vi "Day 8 Task 1.vi"() -> ()   [LabVIEW 2018]
uses:
  <userlib>/_OpenG.lib/array/array.llb/Search 1D Array (I32)__ogtk.vi
  <userlib>/_OpenG.lib/array/array.llb/Delete Elements from 1D Array (I32)__ogtk.vi
  <userlib>/_OpenG.lib/array/array.llb/Remove Duplicates from 1D Array (String)__ogtk.vi
panel:
  out "and the other is f":string
  out "the letter it doesn't have is c":string
  out "6":string
  out "representation of cf":string
  out "representation of eg":string
  out "representation of bd":string
  out "representation of a":string
  out "Found? (index is digit)":bool[][](array[boolean])
  out "no lines":i32
  out "6 digits long":string[][](array[string])
  out "5 digits long":string[][](array[string])
  out "representation of digit (index is digit)":string[](array[string])
  out "0=a,1=b etc":string[](array[string])
  out "sum":i32
  out "tally":i32[](array[numeric])
  out "tally of digits (index is digit)":i32[](array[numeric])
  out "4 unique output patterns":string[][](array[string])
  out "10 unique signal patterns":string[][](array[string])
  out "Tally that number of segments lit occurs":i32[](array[numeric])
  out "Number of segments lit":i32[](array[numeric])
  out "Digit":i32[](array[numeric])
  out "Segments Lit":string[](array[string])
  out "No. Segments lit":i32[](array[numeric])
  # "6"
  # "x"
  # "5"
  # "5"
  # "x"
  # "5"
  # "6"
  # "x"
  # "x"
  # "6"
  # "common between 6s: abfg. Not common between 6s: e(2)c(2),d(2)\ncommon between 5s: adg. Not common between 5s: b(1),c(2),e(1),f(2),"
  # "mapping of a is in digit 1 but not in digit 7\ngot a\n\ndigit 4 NOT digit 1 = bd\ndigit 8 - bd - a - cf (1) = g\ngot ag\n\nfind the letters common between 5s = adg\nadg not ag = d\ngot adg\n\ndigit 4 NOT digit 1 = bd\nnot d = b \ngot abdg\n\ncommon between 6s: abfg\nbf AND cf = f\ngot abdfg\n\nfrom cf got c\ngot abcdfg\n\nwhat's left is e\n\n\nThere are only 2 digits without an a: 1 and 4\n\n\nmapping of g is in (4 and 7) but not in digit 9\nmapping of d is in digit 3 but not in digit (1 + a+ g)\nmapping of 5 but not (1 + d)"
  # "--> occurences of length 2,3,4 and 7 are unique\nCan find digits 1,7,4,8"
  # "the 6 letter that does not have cf is 6"
  # "de is diff the other 2 6s"
  # "the 5 letter with ACF is 4"
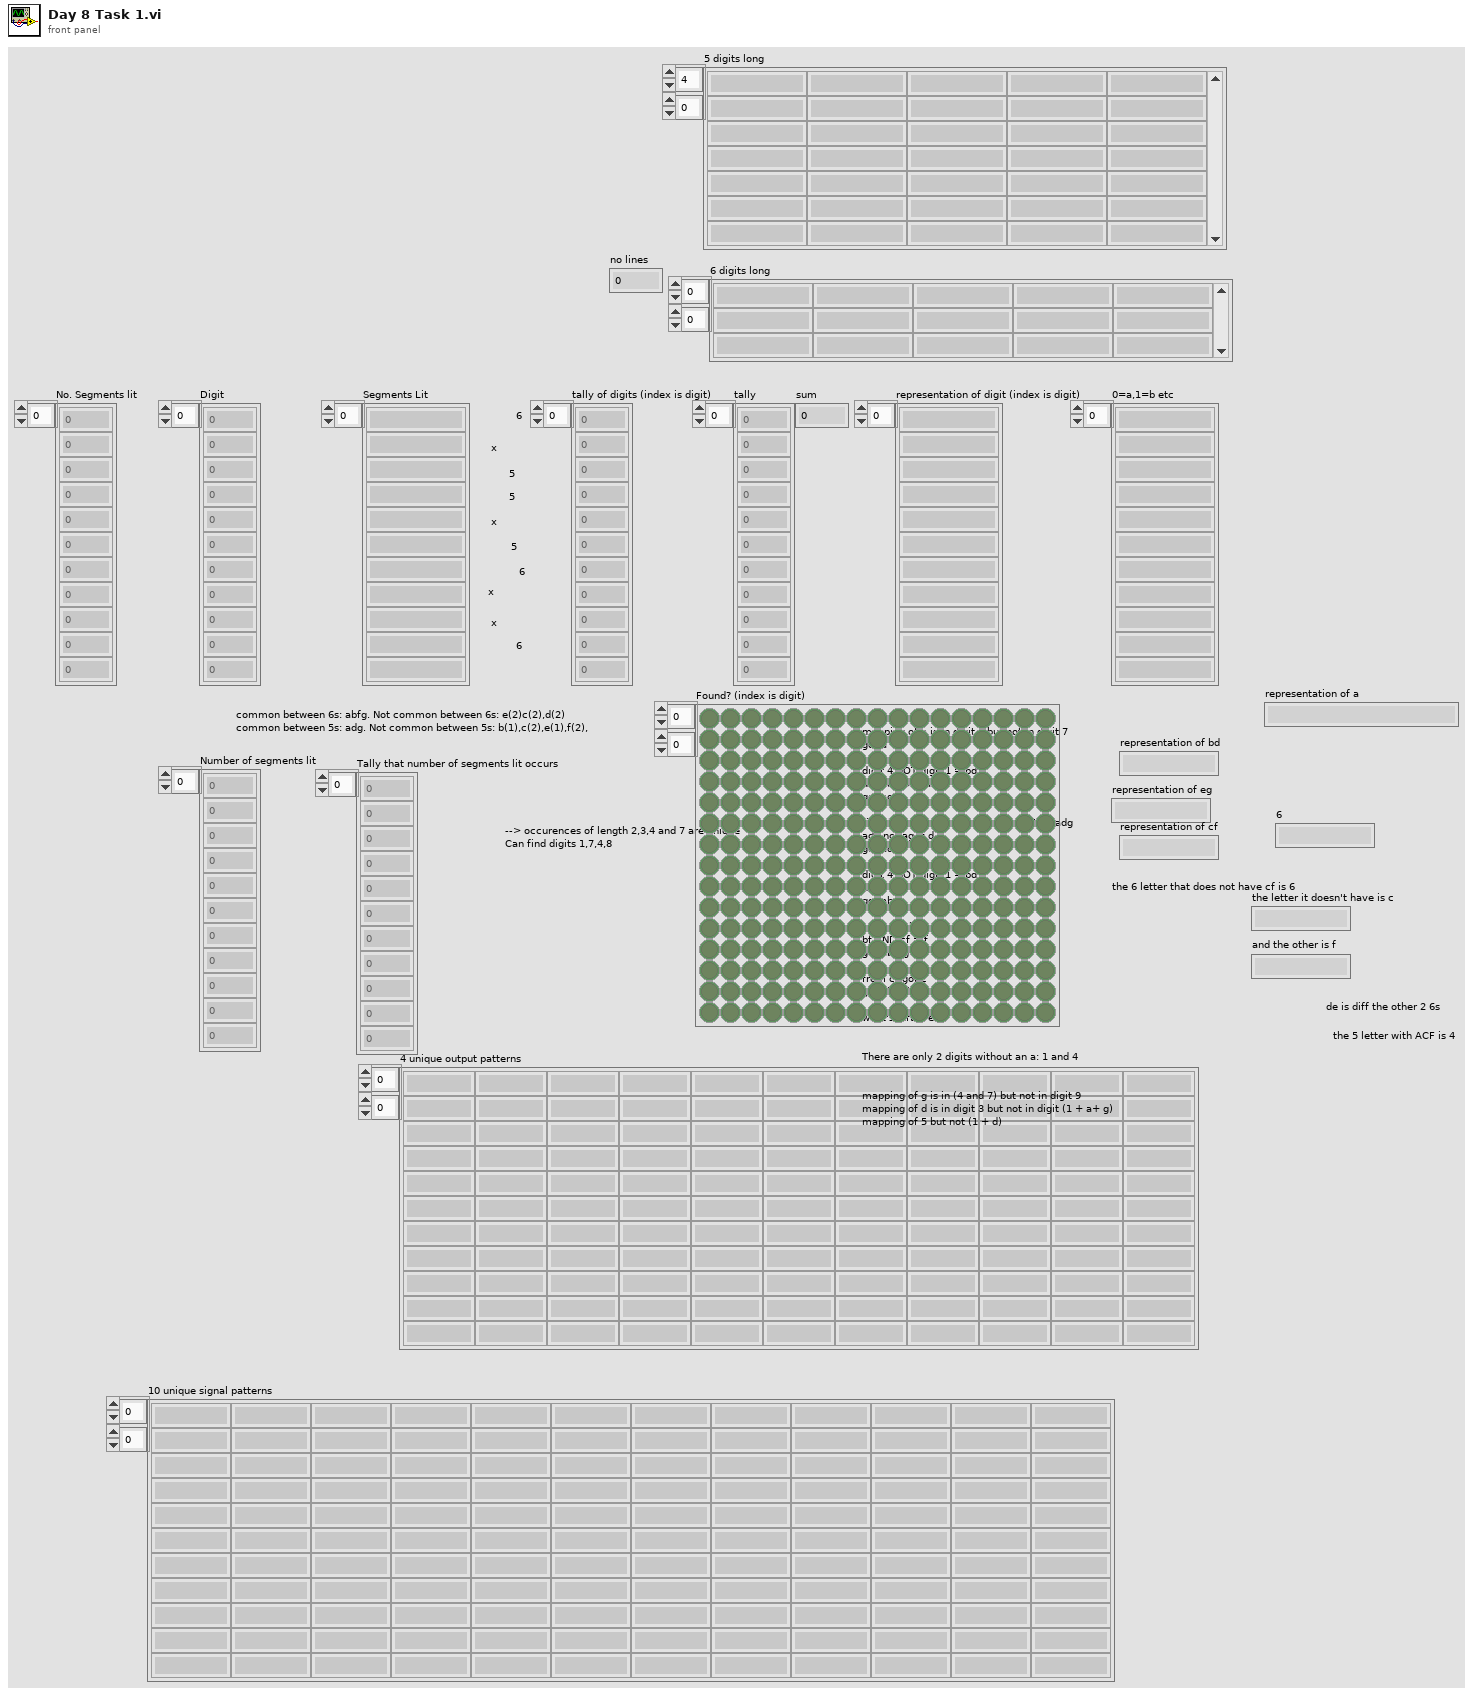
[diagram p1: front panel]
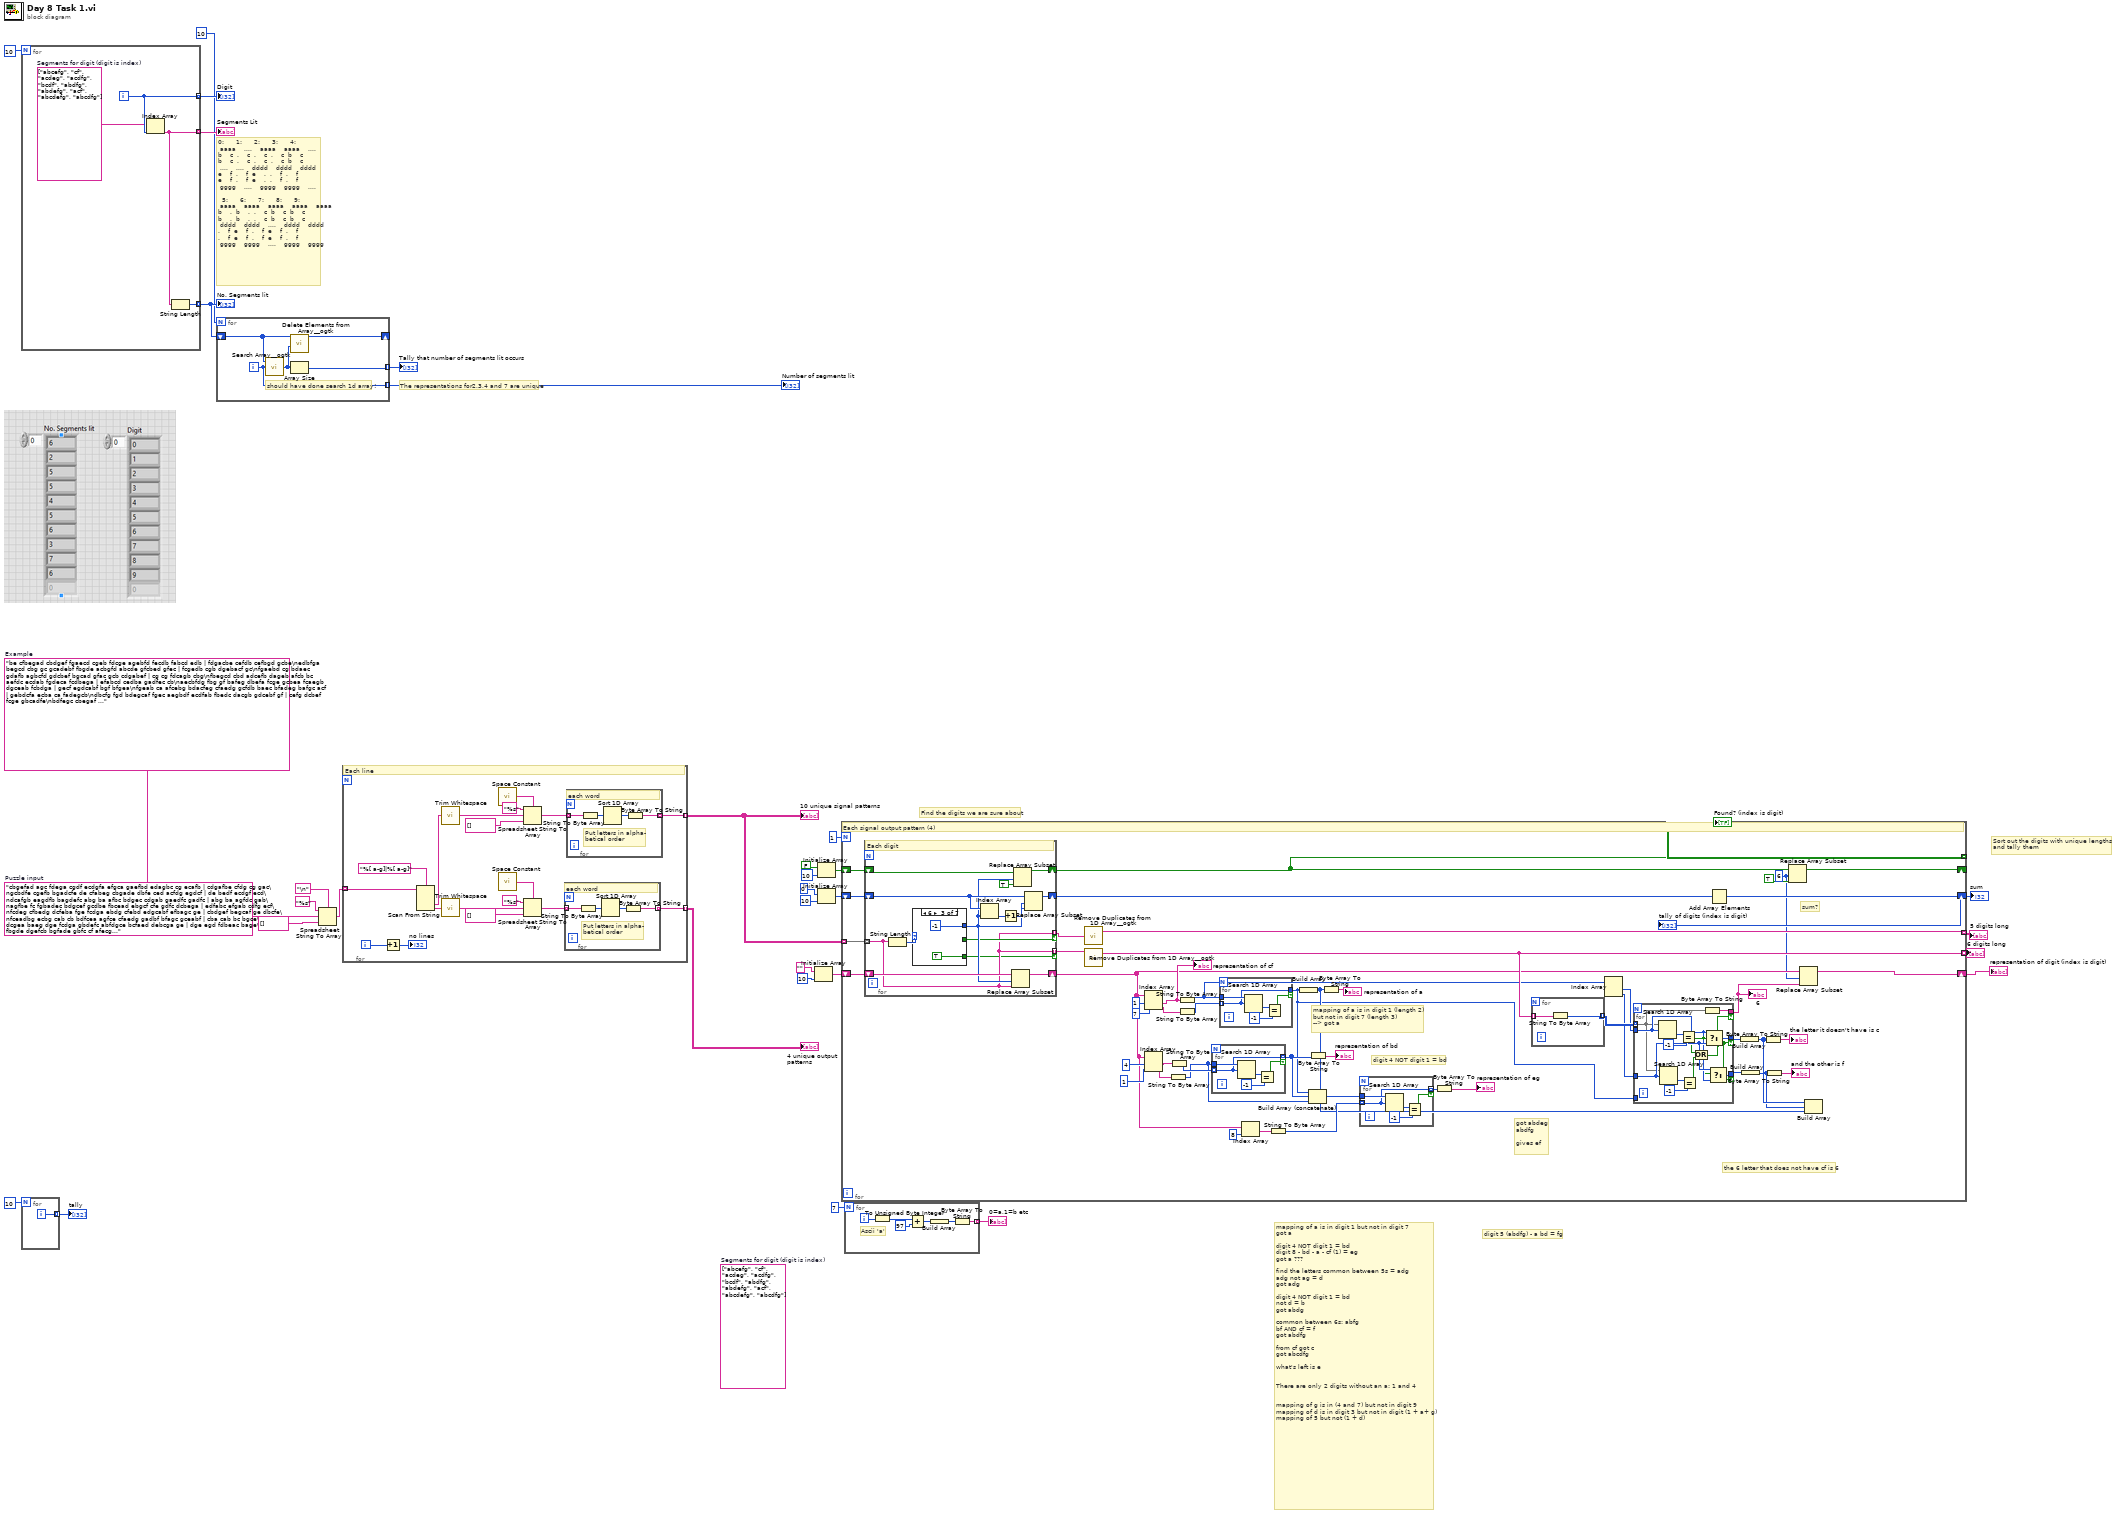
[diagram p0: block diagram]
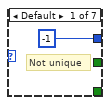
[diagram p2: hidden frame]
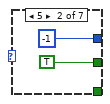
[diagram p3: hidden frame]
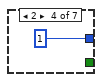
[diagram p4: hidden frame]
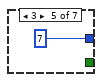
[diagram p5: hidden frame]
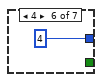
[diagram p6: hidden frame]
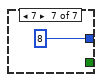
[diagram p7: hidden frame]
diagram:
  (unwired) string[] ["abcefg", "cf", "acdeg", "acdfg", "bcdf", "abdfg", "abdefg", "acf", "abcdefg", "abcdfg"]  # Segments for digit (digit is index)
  (unwired) "cbgefad agc fdega cgdf ecdgfa efgca gaefbd edagbc cg ecafb | cdgafbe cfdg cg gac\ngcbdfe cgefb bgadcfe de cfabeg cbgade dbfe ced acfdg egdcf | de bedf ecdgf ecd\ndcafgb eagdfb bagdefc abg ba afbc bdgec cdgab gaedfc gadfc | abg ba agfdc gab\nagfbe fc fgbadec bdgcef gcdbe fbcead ebgcf cfe gdfc dcbega | edfabc efgab cdfg ecf\nfcdeg cfbedg dcfeba fge fcdga ebdg cfebd edgcabf efbagc ge | cbdgef begcaf ge dbcfe\nfceadbg ecbg cab cb bdfcea agfce cfaedg gadbf bfagc gceabf | cba cab bc bgce\necadb dcgea baeg dge fcdga gbdefc abfdgce bcfaed debcga ge | dge egd fdbeac bage\ndfc fbgde dgefcb bgfade gbfc cf afecgbd cadge fdegc abcfed | cf cfgb dagec bdegf\nedaf bagcdf bafegd efacdbg fbaecg gcbde ad gda bfaeg edbag | dgbafe fcbgae adg dag\nfbgdca efacdb faegcbd egbfd acebf feagb ga ecga bgefca gaf | geca gaf gdefacb egac\ndcfeab adcfb eac dbgace agdefbc ae decfg caefd feab agfdcb | fgecbad cae bfae eca\nbefg bcafe begacd ebgfac eba fgeadbc dabgcf bgcaf eb feacd | eafcb agcfb gcbfa facde\nacefgdb cbadeg gbcde cde dfbgae eagc dfbeac ec bgade dgcbf | cagfdeb ce gafcbed dgcfb\ndafbg cdebg ca cabfge cead fcagbed abcgd febcgd agc egbdac | agc cdebg gac bdgaf\ncfbged bfc egfc eadbc fbacgd gfbde dbfce efabdg efdgacb fc | bfegd fbc fcagdb dcefbg\nbg fedbcg eadgf edagb dbg fgba dgfeab gafcde aecdb dgfaebc | degfa bdg egabd gbade\ncedb fedgbc aedgfb efdgb dagcf cfe ec fdceg caefbg gaebcfd | ec fcgebda dbec dgbfe\nbdgeac fbgedca cg bcedg gcb bcefga gacd dfegb adebc ecbdfa | edcagb cgeafbd agcd dgca\nfa bfa abcfeg bfgea gdabe defcgb cbgef efca cbedagf fcdgab | fa cegdfb bfecg ecaf\ncabfd egbafc bdae dcaef ba gcdfb gcdfae abc bfgdeca daefbc | cfeda eabd gdbcf gcedfa\ngbcdafe cfgdab becf bdf edcbaf bf cebagd bdeaf efdag cdaeb | afdeb febc bf fb\ngebad caed gcbfde befacg dfgacbe dbcaeg gea ea gbafd dcegb | gbecaf gafceb cbagef caedfgb\nadebgf cgafbe agbdc cafbedg dg dcaebg gdb bcadf egabc cgde | ebdgacf cbeadfg fdaegcb bcgdefa\nfcbgae gce bgdfec acgf daefbc eacbg bcaef gaebcfd gc aegdb | eafdcb gbaec cgfa fcag\nbdfgce ca dcfbae ceafgd dgfca abefcgd dgabf acd aceg gecdf | fabgd cda gacfed dac\ngdbfea agcbde abdec dbaefgc fbcae dgeac cdgfae bcdg bd ebd | gcebad adgbef db bd\nadcb acgde cde cd baegc edbcgf edacbg gfdea gfabce edgfbac | defbcg dce bfeagdc gbacef\nafe agcbfe dgbeac af fcebd afgc aebfc gbadefc egbac gabfed | af ebgcfa af fea\nfea cgafbed debga bfgdae fa dgefc aegfd gafb cdafbe dacbeg | af afgde af bcadefg\nfcegdab dabcg gdbaec becd de afcdgb abged eabfg fecdag aed | bacdg aed de ade\nbd gbd gbecf fbcgd egfdab fagdc bdec fegbdac dfgecb facegb | cedb bdfegc gbdface egcbf\ncfagd bdcf bcdgea gcabfe dc cagfbd fdgecba cad bacgf afegd | geacbfd cbdgaf dgbfac cd\ngace fdbeca gba cbfae bgdfca efbag dbefacg bcagfe ga fbgde | adcgfbe ga ag cdbafe\nfb fgecbda dabecg bfedgc gcfbe ebgdc ecfdab fagce fbe dfbg | fb bfcdeg cdfegb bf\ncdge afedbc bgc fdcbg dgfbec ebdfc becdgfa ecfgba cg dgfab | decg bfaedcg fbdag cbfgd\nbdafgc gacdf cafgdeb fcdega dfabge edacf fde ed cged bfeac | abdcfeg de abfce bgdeacf\ncgfbe de cfebag faedbc gbdfe gbcdfe ecgd def dgbfa dfaegcb | decg ebgfdc ed gbceaf\ngfd fcgbd fdgeba df ecdf cdfebg efbcag fbgaecd cgbfe bgdac | gfd efcd gfd dcef\ndafe bcaed dbf gfdceb fd agcfb aefbdc beacdg ebfacdg cfbad | fead bdf abefdc defa\nbgdce facg fgebad efcda gefcd dcfaeg dabfegc cabfed gfe gf | ecadf dgcaebf gdfabec fg\nbcfaed cgeafb cgfedb gcdabef fbecg gacdf facgb abge baf ab | bgae bdgceaf dfcga eagb\ndegcbf bec aecgdf acdegfb fcbd dgaecb fegab fgdec cb cbefg | gbeaf dfcb gbfdec adcfgeb\ncgef cbeafd bgafed ec gefdabc cae deagf caedg cgbda feadgc | ce feabgd ecgad efcg\nfgdbae geabcdf ega fdecg ea acbe cbagf cegfa fbagdc aebfcg | ae gea acbe ceab\ngabe dcfbae ae dgefc dea cbafgd gebdaf dbgfeca gbadf gefad | ade aed ead adefgb\nfabdc cgbdef gdec aecgfb bgfde ebcfd afbdceg ce cef egbafd | cdfbge dgce cabgef ce\nebfacg gdce gbefcd befgd cdabf cfdgb cg efbadg bcg aebgdfc | gbfdc gcb dcge bdcfa\nefagc geadfb ca fegcad fca defabc fbgec egfda dgac cbedafg | cdag caf caf dgac\ndbaec bd efcda dagcfeb adb cgbea cdgb dacgeb aegcfb baegfd | bda efbcgad cdbg gacbe\nge acbge bedg aeg agfdec cabgd bcdgfa edgcafb egbcad befac | gecba ge fcgdae cdbefag\nfdbae gacfde fecbd cgdfeb af gaebcdf aef bfca gaebd cafdbe | aef fea edcgbaf fcbed\ndcfg bfagd cdebaf cbaeg fcagdb bdgaef gfacb dfcgbea fac cf | cfbgeda debfga gaecb cf\nfbdaec bdfca gd bfgcd gbd bedgca gbefc abdgcf gadf gcdbfae | cdefagb bdg fcabgd dg\necbgafd ecdgab abedfc eafbgc cabef abd da fcad baedf fgbed | cbeagf dba faecbdg ad\nbdefg ecfbd ec cfe aebc fdgeca cbadf cagfedb fbcagd efbcda | ecf ec ec efc\neadfcgb gebdfa afcdb agefd adgbf bgea gb adfecg gfbdce fgb | gbea gbf gcfdeba ageb\ncb fegba dfcbgae gefdc gebfc fadbec cbe agfbec adgfbe cbga | daebfc abgc egcdf ebc\ndgfec dg bfadcg gacfde eafgcdb agde agcfeb cebdf cafge cgd | bcedf dg dg abdecfg\ngbf cagedbf gadf gcbea ebcfda afbcg afdbgc bfgdec adfbc fg | gfb gdfa fdacb fg\nbd bfd degaf bedaf gbacfd cfaeb ebdfga fecgda acdgebf bdge | eafcb bd eafdgcb bd\ngefba dcagefb gebfad baecf cegbaf fc dacbe fcb egdcbf gcaf | efbga fgca cgadefb dcbefag\nedgaf eagfb bfeagc ed cagfbde gdafc egadbc edfb dge gfbead | gabdcef fdage agbfec dfbe\nagdbfe gd dbeag acgbedf cdbfag gda cfgeab edfg beacd bgafe | gd efdg gbefa agd\ndfgbac efgabd edg afcde bgfda eg abecgfd deagf eagb dbfecg | bedcfg dcbfaeg egd ged\ncdfaegb bdcg bcafde deabg dcagef dg badce gfaeb agd edbagc | geabd abced dga dg\nfaedc bgaec gf cagfe daecbf egcfda fcgd efg cfdbeag bgefad | fecabd afcde gcdf eagdbfc\nbcdgfa eabfd cfbde gcbed cbf efbadc gfdabe gbfdeca faec fc | cfb dbgec dbgec feac\nfgacb abgefdc feacd bdef dbc db bcedag adecgf acebfd fbdca | cbd cbd bd dfbe\nacfdbe daeg gaebfc fga gdcfb dcagbef bfagd ag gdefba badef | ga fadbg agdfb gaf\ngbefdc bfegad feag dae gfebd ae dafgbec dfabe daegcb cadfb | daegfb bdagec ea egaf\nbcage gefadb cfga fbdecga gdbcef bga aegcbf bdeca gfbec ag | ebacg bedcgfa ebgcdf agb\nbdegf dbaegf efabg ag gade fga cedbfg ebfac afcbgd bceafgd | aegfcbd gfdeb bgefdca gaf\nefcadgb dfb bgcad fd fdcbg gefcb gfaecb fdec edbgfc aefbgd | df bcdag fbaceg fd\nfebgcd fgbdcae fdegab cgabf gbfcd gecaf bdcagf cdab bga ba | ba gafdbc gba ab\ngefba dafgb gfcae bfde gdceab badgef be afgbced ebg cfgbda | eb eb fcega deabcg\ncbfdae egabdfc eacbdg ecdab gce agfbc gaed eg gcfbed egabc | gead dbfgace dgebcfa gade\nbacgfd dgfe fdagecb cgebdf fbedc edb eabfc bacdeg fdcgb ed | de ebd dfge debfcga\ndcgae ef bgefda dfabec ecdbgfa acdfb efa fadec cbef bacfgd | cfabged acfgebd dfcba eagcdfb\ngbfde fcd agcedf cdea edgcf gefbac begdcaf gafec gabdcf dc | dc agfec bgedf bfegac\ndebgfa cfgba bag fcdgb bcad ba fedcbg afdgbc eafcg cgfdbea | dcagfeb ba ba bfdcgae\nbfdgae bdfcage edagbc eagbd febac fgbcad cdeab adc cedg dc | gebdfa edcg ebacf ecgd\ncbfdea fcbgade egabd gface bfecga deafcg acegd dc cgdf dca | fcdg fgcd cgfea cgdf\neafcdg cb bedca cdgabfe aefbd gdcea facegb edcabg bac dcbg | cdgb decba gfceda bac\ngbdecfa ceabfd edfgb gfba bgdcfe af dgfeba dgaef fae eacgd | dgabfe fa fadeg gbaf\ndcaegb gdcfea eadcfb dafcg daecg afd gafe bedcgaf bfcdg af | acdfgbe dfa afd fgea\ncfgbdea bfade afecbd faedg bdac aeb fedcb faecbg ba bcgfed | cfdeb egcfdab abe ba\nfgcabd geadbcf cdbe ebgdf feacgb cgfeb db gdebcf dgaef bdg | efbgcd gbadfc ebgdfca dgabcf\ngebfda ge cbfdega cgde gacfe afecb gef bcgdfa cadegf fdgca | ecdg cedg fcgedba abecf\nadebc dbgc abefcd agfde egc gcaebf agecd cg ebafdcg degcab | fgade ceg bgdc gbcd\ngacedbf ebgf afegcd beadf cdeba aebfgd fab bgafcd edagf bf | fbge fgcead debac fegb\nfcgdeb bgdeca gfeacdb edbga gfea fadbg fg aegfbd fgb fbdac | gf gafe caegdb afcgdbe\ncdfeg bd dbfe acdfeg dbfcg dbg afbgc dbgace gdcebf ebcagdf | fcgdb dgb bfcgaed febd\nbecagf dagefc cdebf gefab dgf gfbde bdegfa dabg gd ecfbgda | gd bfadeg gdf fdg\nfcaebg fbadec edgbc fc fagc fec egafb efcbgda fegadb bgecf | fc eabdfg acfg deafbcg\nbe fbgca fbgade fdgace bcde edbgcf cfgeadb degfc ebf bfceg | cbfdgea bcgaf fcegd gfdeba\ncdgba edbgc geca bge gbadce gdfbae dcefb dcfabg gecadfb eg | eg fdbaeg ge geb\ncdbfg ad afegcdb ecfba cdfab adec geafbd cfedab dab bgaefc | cbgdafe faebc da ad\nedbcf cbgedfa gceb eg gfbad egf gdfbec fabcde bfged gefdac | ebgcdaf ge dgcfeb dbfce\nfde fegcba ecdfb acfebd beacf fcdbaeg df afdb bcegd gedfac | gecfba eacfb df cafegbd\nedbafgc gd adecb dfga bgdfae bedcfg geafb aegbd gde cebafg | deg gefbcda dgaf edg\ngfb eagf cdbfae fg gadbf gdcba dabgef fecgdb dfcaebg afdbe | cabegfd cbdefa gfb bgf\ngfa edgfa caefgb gf gbcaed gdcf egcda eabfd edgfac fbecgad | fg fag fg fdcg\ngf ebgda cabedgf gcfb cdfbae gef efcab decgfa ecbgfa abfeg | bcgf gf egf gfe\ngdae ecfbag badgc ebcfda cbgfd gaefdcb ebgdca ceabg adc da | eacgfb bgadc dca cda\nacgbf ceagf cbgafe bfc gbdcfea fdecab bf befg eadcfg dabcg | fdaceb cbf bcf bfge\ncedgb bfe efbcg ef acfe fdbacg cdbgeaf gdbaef gebacf cfbga | bagfdc fbceg cafdbg cagebf\ndbcgae gfbda ca cbdeg dcgba abfgdec acb efdbgc daec bafegc | agecbd dagcfeb ac ac\nbgcfeda gfcba gfe ef degafb eadgb bedf afgbe bdecga gfdace | fe bfde gebaf dceabg\ndefcba facgeb de cbdea ecfba ebdgaf fecd ade bgfcaed cdbga | dea de acebd ed\nbad cgbadfe ecadf ebdcg aedgfb ba aecbd decabg bacg gbfecd | bagc cbag agbc eafdc\ncfgde afgeb aec bcfdae gbac abcdegf agdfeb ca gaebfc aegfc | dafgbe eac bgac facegb\ngecda eb cbdea cdbfa egadbfc fdecag deabgf bde acdebg gbce | cedagfb gceda facdegb ebd\nbgd db fbed fabdg eacdfg dgbecaf cafgb edgfa aebdfg gdaebc | db dfgaec ebdf agdbf\nfgecadb abe cagfbd bcdage eb eadgbf dcfea deafb bfeg agdfb | daecgb agfbdec be gbfe\ndeabg bef caebgfd fdaeb gdebfc fe fcbgda ceaf bacedf bfacd | fe afcgedb eadbf gacbdef\nac gcae aebcd bedcg eadfb bfcged gadcbe acegbfd bac fbacdg | fbgcead cdgbefa dbgcaf bfdcge\negcfa cef cgeab abfc gfedabc abcefg agbdce cf eafgd dbfegc | abcf dafeg fcgbde gaebc\nafdceg dgbec egdca bc cedfab ebdfg bacg ebcfagd egacdb bdc | abgc ecgadb abgc dbcaefg\ncgefab efcd fcg dfcbge dabgc egbfd bgfcd fc dabegf bedafcg | dgfeb fecd fc cf\ndea abcdfge abfecg de edfc ebfac gbcda eagfbd fdaceb daceb | cdgba dbacg badcegf edcf\nabgfd fbaegd bfdcga fgbea agcdebf ge gbde cafgde fge ceafb | ebdg gedb cafegd cbdgfa\nadbg fecbg caegd bcgead ba aecgdf deabfc cbaeg ceafgbd eba | efgdac becfad fcadbe febcad\ncefbag eca cdbeaf dbcefga fbdca dgbcfa efdag decb dfeac ce | cgbaefd ec aefdg cea\nbdgfae acgeb cegfd egdca efcdbg dcfa ad gda cgafed cdgabef | ad acedg ad fgdecba\ngdfa dcg bcegad gd bfaecg afdcge cedbf cgfae gfedbca fcdeg | gcebda gcd fbedcga cdg\nebafgc da fbdag fgbca bagdfec gdfeb cgfabd dabc egfdca gad | ad badc dagcebf fecdgab\nabd bdagfce adfceb adbcf egbfda febgdc da cead acgbf cbedf | bgadef efbcdg da fagbed\nbae dfagbe fecba edacfbg baecdf bdec gbdcaf be bdacf agcef | ecfadbg be abegcdf bdec\nbcd fegadb gcafebd badgec eadc abdfcg aegbd dc gcedb fcegb | dbc cd abdgcf acgedb\nfg bfdeg dfeab dfg cbegfd ceadbg efadgcb cdbge fgce dfgcab | gbafecd gfcbda gfd bdgaec\nagcf acb edfgcb fabdcge begad ac dfgcab dgcbf abdgc cebfad | gfedabc badge gacf ebgda\ndfgabe fge dbfagc edfca gebc ge badgecf fagec fbgac baecfg | cegfa gfbca fcdbga eg\ndagb ebgdf fgbaed ab ecbfadg befga fabcde baf fcega begdcf | gbfcaed afb adbg bgda\ndfgec efabcg ebfag cga agbdef beac dgfacb cagdbef ca fgaec | ecbgaf fagce cag bace\nae fgbdea dbcfag cbea begdcaf gea gdecf decga cgdabe bagdc | ae ega bcfagde ae\nbgaec efgbadc cgeafb becdga cadbfe bafgc afeg fa bfa fgcbd | fdabegc afb feag gbace\ncfbdgea egfabd ed afecg fdaec cdafb cgdafe dae gfebca cged | cagfe cgfbade ed dceagfb\nbfegad ecdb acbfg gdb fdcgeb db bdgfc acebdfg cdgef dcfgae | gbd bd cdeb gcefd\ndcba cb decfga bagfe gdabecf bdgafc gcdfa bgc ecdfbg abgcf | bc gdaefc fcdeabg fbage\ncf efdc cdfgba dcgaef dbegacf fgbea ecgfa ceagbd cfg decag | gedcab cf fedc cf\ncg gadcef edabcgf dgfea abefgd ebgdcf acfge cge baefc cdag | gc begfda gc gedaf\nbc fcageb cbg cfagd cfgdb agcfed fdebgca dcfbag efgbd bcda | abcfge fgdeac bc bcda\ncgabf cf efdacgb cgaeb cefadg bcefga fgc ceagdb ebfc badfg | dbfga gcf gacbf cbegaf\ndbg cfbgae dbceg cagd gd gbfdeac cgaeb bfecd agfebd decabg | eacbgfd eadgbf dg agecbd\ngebfdc gcabf bdcgfea gcdba fcdgea afbe cafeg bf fbc beagcf | fbae agfbc cbgefad afgcb\nfcae baefdgc feadcb cedba fbe fe bagfd bdefcg edafb abedgc | faec dcegba dagceb fgdba\negfbcda ecbfg ebdcgf fcadbg cd ebdc edcgf gafed efbcga gdc | bced bdgcfae dgfec efabgc\ngeb gfdeac feagc egbfc dbcfgea cebfd fdeagb bcfega bacg bg | abcg cbag bge dacbefg\nbcdef afe ecab bcefdg edfca febcad ea cfagd dfbegca dagbef | ea fgdeab afe eaf\nacdbegf gbcfda bfge dcefb bgd febadc dcaeg gb degbc gfdecb | fabcdeg aecgd gbd gb\nfba cdaefb cbgefd ba afebdg afegb bgacfed fbdeg gbda caegf | ab efdgb bgad dfebg\neaf bcegda fe gacef gefb agcbe cedfbag dagcf defbac afecbg | ef aecfg ebgf gbedafc\nfgedb ad fcage dcae cedbafg aegdf dagefc afd gafcdb geacbf | gcaef befagc da dfbgaec\ncbdga ecb bcade dgaceb dbeg cbdfag eb fcagbe gebcdfa dface | edbg begd dcbea beadcfg\nbadfeg af egcdbf deacbf dbacf abgdc dfbagec fba cdfeb afce | cgbad dbgfae fcbad acdefb\ned ced cfaebdg deaf bcgfe bgadec dbafgc dacbf defacb dbfce | afed bgcaefd cgbef gafedcb\ngcfba cbdgea aecgdf cdgebf be bec gcbea dbae gacde egbcdfa | agcbf dcgabfe fagbdec ebda\nfedbag fagcd dagfe efgc faebgcd egabcd cag badcf fagcde gc | agdfc caedgb gca cg\ngbfecad bdafge fgb bfdae eabfdc fgbeac gcdfa bg debg bgdaf | febad fgceab dfcaeb bgf\neb ebd dgcabf gcabde fcedgab aebg cgadb abfdec ebgcd cfdeg | ebgcd cbfgead bfedgca deafbc\ned acdgfb aed gefabd fegcabd gfed bdaegc edbfa bfeca gdfab | aed ade fdgbace fgadb\nbg bfecad fbg bedgcf agfdc efdcb cgbdf bceg fgebcad beadgf | bfg bcgfd dcegabf febdac\ncd bgfadc befcga bfcga gacd ecfgdb dfabe dfc bfdca fcgbdae | cbagfd cfd cabfdge dcbfga\ngae cbfega adbef acebfd geadb dagbc adgefb ge egfd fcgbead | eg fbegacd edgf eg\nfdgbaec abfc gebdfc fa afgbe bfceg dbage cebfag gaf egcafd | cfba dageb afebg fcagbed\nacfeb ab bdae afb cbfdga fcdae aefcdg ecfgb cdeabf dfgcbea | abf gdabfc dbefac bafdcg\ngcadf febgac gfcbed bcgdf gfa dacfe ga ecfagdb cfbgda abdg | agf edfca egcdafb fag\ngef cbfeag cafg gcbae edabcg dfaecgb fg dafgeb ecfbg fdceb | cafg fg ebfcag ebcfg\nfaedbc fb egcdf cagedb bcdfg eacbgfd bdgac bfc gcadbf afgb | fcedbga bdcag fb aebcgfd\nafdeb cafeb becgdfa fgce gcabfe fgcab bgcfda ec bdegca bce | gdcfaeb dgbecfa adfgbc bce\ndcega fdgaec aegb bdgca gafdecb fcdab cefdgb egbdac bg gbc | bg bcg gbae bage\ncabedg aedbf dba gbdeaf gfba decgbf ab gadfbec edcaf egbdf | eafbd gabf fgba ba\ngbcda daegfcb efadb fg cgeadb fcbeag agbfd fbg dfgc bfacdg | dabcgfe gcdfba gbcade acgfbed\nbgcda gd fagd bdacfge abgec acbfd agdfbc acefbd gdc gbdefc | dg adbcfg beadfcg gbcda\nfgbd cbf bcdfag bfgca fb cfgaed abcge cgafd cdfbae bdgceaf | aegcb fcb bcf bf\ndaebgf cbefdg cdegfa adce ad fdecbag dgcfe gcbaf gda gdacf | cfgba gad da da\ncagdfb egcbfda fbadc gdc efcabd cbfgd efgcb dgeabc adfg dg | cgd dbefgac fdgabce agfd\nfedcag gadfceb abecfg cgdbe fcedg gafedb fc deagf dcaf cgf | fc fgc cfda fdac\ndgcafe befg fec bcgdf ecdba afgbcd ef cefbd aedfgcb bdcgef | cbead gbfe agdcbfe ecf\ncedbaf dcbfa cfgedba gdcbf fecbga daec ad fgedab faceb bda | dgaefb cead fecdgba bafdec\nbcdef fgebac fdgb fb edcbgf fbc fagdec fcgde abfgcde cebad | bdfaceg fbcdgea fb bdfegc\ndcbea fegdba gaedb cbgdef bg egb fagb feagcd dgafe fdabcge | dcaefbg bfga gafb gfdeab\naecgfd debagc dbgfa dab edabgfc cdafg fbca ba gfbde dcbgfa | ab abdegcf ecabgfd ba\ncdefbg fcabd cega bdafeg ag begdca bdagc egbcd dgecfba abg | gbfeadc aceg ag egca\ngbfcade gecfa fdceag bdefa bcag gb gfb eafbcg dbgfce faegb | gcab gb bfade cefbdg\nfe acdbf gbeafd dafgcb afbce dgfbeca dcef efa gcbae dfcbae | afe cgeba ecdf fbeadc\neacd gdc acfdeg begdfac cfdga agefd bcgfa bgefdc fegadb dc | cd cd dabegcf ecfgabd\ncde dabfc eagbd abfcdg bedca afdcbe cfeb daegfc cfegdab ec | ce ecd adcfb gaedb\nbedacf fc gfedb fecgadb gcdafe degac dfgce cfga cdf cgdeab | gcfed bgfed ebdfg cdf\nafdbce gcfadb fg dgcae bagedfc fegca ebfg eafgbc fag abefc | cafbgde gf efadcb fgbe\nfgbedac agcbe cegbf cbfdg bcgaed fgebda ef acfe bfe gceafb | egacfdb ef cabfeg ef\nadegb bcaedfg deaf fa afb gcefb edbcag efbgad afgbe bagcdf | edbag fba af dgabefc\nedgabf aedc fbagc da ecbgdf bdcga agefdcb gad ecdgb cbdega | cbdag ad fgbdcae dbceg\nec gecbfa cagedf fadge fbgeda cbdga cfde eacdg ceg cfgaebd | ecg ec ecfd ec\ngcafeb egbdc bdac daceg dbfge bc cdafge ebc cgdeba fabdgce | dgcbea dfcabeg gdfeca cbdaegf\naeb edbgcf ba dbcge adbg cbgeaf bceadg faced cbaegfd deacb | dfeac bea cebgfa ab\nfgacb gdeafb fegabdc bfagec cgf dcbaf ecgfad cbeg cg afebg | gfc fagceb cdfgae fcg\ngb gdb gbca ecfgbad cdfgbe afcdgb dfbga bfead gcafd feacgd | beafd bdg dgb aefdb\ngb caebgd gfcb aegdfcb acfbe edgaf abg bgfea beagcf dcefab | bga dafge agbdefc efabgc\nfebcga bfgcda afc cbagefd agcd bfecgd ac dfbca cbfgd befad | ac fca afc cdfab"  # Puzzle input
  w3 = "be cfbegad cbdgef fgaecd cgeb fdcge agebfd fecdb fabcd edb | fdgacbe cefdb cefbgd gcbe\nedbfga begcd cbg gc gcadebf fbgde acbgfd abcde gfcbed gfec | fcgedb cgb dgebacf gc\nfgaebd cg bdaec gdafb agbcfd gdcbef bgcad gfac gcb cdgabef | cg cg fdcagb cbg\nfbegcd cbd adcefb dageb afcb bc aefdc ecdab fgdeca fcdbega | efabcd cedba gadfec cb\naecbfdg fbg gf bafeg dbefa fcge gcbea fcaegb dgceab fcbdga | gecf egdcabf bgf bfgea\nfgeab ca afcebg bdacfeg cfaedg gcfdb baec bfadeg bafgc acf | gebdcfa ecba ca fadegcb\ndbcfg fgd bdegcaf fgec aegbdf ecdfab fbedc dacgb gdcebf gf | cefg dcbef fcge gbcadfe\nbdfegc cbegaf gecbf dfcage bdacg ed bedf ced adcbefg gebcd | ed bcgafe cdgba cbgef\negadfb cdbfeg cegd fecab cgb gbdefca cg fgcdab egfdb bfceg | gbdfcae bgc cg cgb\ngcafb gcf dcaebfg ecagb gf abcdeg gaef cafbge fdbac fegbdc | fgae cfgab fg bagce"  # Example
  # "digit 5 (abdfg) - a bd = fg"
  # "mapping of a is in digit 1 but not in digit 7\ngot a\n\ndigit 4 NOT digit 1 = bd\ndigit 8 - bd - a - cf (1) = eg\ngot a ???\n\nfind the letters common between 5s = adg\nadg not ag = d\ngot adg\n\ndigit 4 NOT digit 1 = bd\nnot d = b \ngot abdg\n\ncommon between 6s: abfg\nbf AND cf = f\ngot abdfg\n\nfrom cf got c\ngot abcdfg\n\nwhat's left is e\n\n\nThere are only 2 digits without an a: 1 and 4\n\n\nmapping of g is in (4 and 7) but not in digit 9\nmapping of d is in digit 3 but not in digit (1 + a+ g)\nmapping of 5 but not (1 + d)"
  # "Find the digits we are sure about"
  # "Sort out the digits with unique lengths\nand tally them"
  # "The representations for2,3,4 and 7 are unique"
  # "0:      1:      2:      3:      4:\n aaaa    ....    aaaa    aaaa    ....\nb    c  .    c  .    c  .    c  b    c\nb    c  .    c  .    c  .    c  b    c\n ....    ....    dddd    dddd    dddd\ne    f  .    f  e    .  .    f  .    f\ne    f  .    f  e    .  .    f  .    f\n gggg    ....    gggg    gggg    ....\n\n  5:      6:      7:      8:      9:\n aaaa    aaaa    aaaa    aaaa    aaaa\nb    .  b    .  .    c  b    c  b    c\nb    .  b    .  .    c  b    c  b    c\n dddd    dddd    ....    dddd    dddd\n.    f  e    f  .    f  e    f  .    f\n.    f  e    f  .    f  e    f  .    f\n gggg    gggg    ....    gggg    gggg"
  n1 = for {
    N: 10 -> [_]
    tunnel: [w38] -> w32 mode=indexing
    tunnel: [w36] -> w33 mode=indexing
    tunnel: [w35] -> w31 mode=indexing
    i -> [w38]
    w37 = string[] ["abcefg", "cf", "acdeg", "acdfg", "bcdf", "abdfg", "abdefg", "acf", "abcdefg", "abcdfg"]  # Segments for digit (digit is index)
    n2 = Index Array(array=w37, index=w38) -> (element=w36:string)
    n3 = String Length(string=w36) -> (length=w35:i32)
  }
  "No. Segments lit" <- w31
  "Segments Lit" <- w33
  "Digit" <- w32
  n4 = for {
    N: 10 -> [_]
    tunnel: [w39] -> w20 mode=indexing
    i -> [w39]
  }
  "tally" <- w20
  n5 = for {
    N: 10 -> [_]
    shift-right: [w43] -> _
    shift-left: w31 -> [w44]
    tunnel: [w41] -> w30 mode=indexing
    tunnel: [w40] -> w28 mode=indexing
    i -> [w41]
    # "should have done search 1d array!"
    n6 = call-poly <userlib>:"Search Array__ogtk.vi"("Array"=w44, "Element Data"=w41) -> ("Indices of Elements"=w42:i32[])  [unwired: 7 in]
    n7 = call-poly <userlib>:"Delete Elements from Array__ogtk.vi"("indices"=w42, "array"=w44) -> ("array w/ subset deleted"=w43:i32[])  [unwired: 8 in, 1 out]
    n8 = Array Size(array=w42) -> (size(s)=w40:i32)
  }
  "Number of segments lit" <- w30
  "Tally that number of segments lit occurs" <- w28
  n9 = Spreadsheet String To Array(delimiter (Tab)="\n", format string="%s" ("spreadsheet string"), spreadsheet string=w3, array type (2D Dbl)=string[] []) -> (array=w27:string[])
  n10 = for {
    tunnel: w27 -> [w62] mode=indexing
    tunnel: [w49] -> w5 mode=indexing
    tunnel: [w47] -> w4 mode=indexing
    i -> [w46]
    # "Each line"
    n11 = Increment(x=w46) -> (x+1=→"no lines":i32)
    n12 = Scan From String(format string="%[ a-g]|%[ a-g]", input string=w62) -> (output 1=w54:string, output 2=w51:string)  [unwired: 4 in, 3 out]
    n13 = call <vilib>:"Trim Whitespace.vi"("string"=w54) -> ("trimmed string"=w53:string)  [unwired: 1 in]
    n14 = call <vilib>:"Trim Whitespace.vi"("string"=w51) -> ("trimmed string"=w52:string)  [unwired: 1 in]
    n15 = call <vilib>:"Space Constant.vi"() -> ("String"=w60:string)
    n16 = call <vilib>:"Space Constant.vi"() -> ("String"=w55:string)
    n17 = Spreadsheet String To Array(delimiter (Tab)=w60, format string="%s", spreadsheet string=w53, array type (2D Dbl)=string[] []) -> (array=w50:string[])
    n18 = Spreadsheet String To Array(delimiter (Tab)=w55, format string="%s", spreadsheet string=w52, array type (2D Dbl)=string[] []) -> (array=w48:string[])
    n19 = for {
      tunnel: w48 -> [w64] mode=indexing
      tunnel: [w63] -> w47 mode=indexing
      # "Put letters in alpha-\nbetical order"
      # "each word"
      n20 = String To Byte Array(string=w64) -> (unsigned byte array=w66:u8[])
      n21 = Sort 1D Array(array=w66) -> (sorted array=w65:u8[])
      n22 = Byte Array To String(unsigned byte array=w65) -> (string=w63:string)
    }
    n23 = for {
      tunnel: w50 -> [w68] mode=indexing
      tunnel: [w67] -> w49 mode=indexing
      # "Put letters in alpha-\nbetical order"
      # "each word"
      n24 = String To Byte Array(string=w68) -> (unsigned byte array=w70:u8[])
      n25 = Sort 1D Array(array=w70) -> (sorted array=w69:u8[])
      n26 = Byte Array To String(unsigned byte array=w69) -> (string=w67:string)
    }
  }
  "10 unique signal patterns" <- w5
  "4 unique output patterns" <- w4
  n27 = Initialize Array("" ("format string"), 10 ("dimension size")) -> (w13:string[])
  n28 = Initialize Array(FALSE, 10 ("dimension size")) -> (w10:bool[])
  n29 = Initialize Array(0, 10 ("dimension size")) -> (w21:i32[])
  n30 = for {
    N: 1 -> [_]
    tunnel: w5 -> [w118] mode=indexing
    shift-right: [w116] -> w19
    shift-left: w21 -> [w117]
    shift-right: [w83] -> w12
    shift-left: w13 -> [w115]
    shift-right: [w85] -> _
    shift-left: w10 -> [w114]
    tunnel: [w91] -> w7 mode=indexing
    tunnel: [w92] -> w6 mode=indexing
    tunnel: [w84] -> w2 mode=indexing
    w81 = 6 ("index")
    # "the 6 letter that does not have cf is 6"
    # "sum?"
    # "digit 4 NOT digit 1 = bd"
    # "got abdeg\nabdfg\n\ngives ef"
    # "mapping of a is in digit 1 (length 2) \nbut not in digit 7 (length 3)\n--> got a"
    # "Each signal output pattern (4)"
    n31 = for {
      tunnel: w118 -> [w150] mode=indexing
      shift-right: [w158] -> w116
      shift-left: w117 -> [w159]
      shift-right: [w157] -> w82
      shift-left: w115 -> [w156]
      shift-right: [w155] -> w84
      shift-left: w114 -> [w154]
      tunnel: [w150] -> w113 mode=indexing if=w151
      tunnel: [w150] -> w112 mode=indexing if=w149
      # "Each digit"
      n32 = String Length(string=w150) -> (length=w162:i32)
      n33 = case shown="6" w162 {
        tunnel: [-1 ("index") -1 ("index") -1 ("index") 1 ("index") 7 ("index") 4 ("index") 8 ("index")] -> w153
        tunnel: [_ TRUE _ _ _ _ _] -> w151
        tunnel: [_ _ TRUE _ _ _ _] -> w149
        frame Default {
          # "Not unique"
        }
        frame 5 {
        }
        frame 6 {
        }
        frame 2 {
        }
        frame 3 {
        }
        frame 4 {
        }
        frame 7 {
        }
      }
      n34 = Index Array(array=w159, index=w153) -> (element=w161:i32)
      n35 = Increment(x=w161) -> (x+1=w160:i32)
      n36 = Replace Array Subset(array=w156, new element=w150, index=w153) -> (w157:string[])
      n37 = Replace Array Subset(array=w154, new element=TRUE ("new element/subarray"), index=w153) -> (w155:bool[])
      n38 = Replace Array Subset(array=w159, new element=w160, index=w153) -> (w158:i32[])
    }
    n39 = call-poly <userlib>:"Remove Duplicates from 1D Array__ogtk.vi"("Input Array"=w113) -> ("Output Array"=w91:string[])  [unwired: 1 out]
    n40 = call-poly <userlib>:"Remove Duplicates from 1D Array__ogtk.vi"("Input Array"=w112) -> ("Output Array"=w92:string[])  [unwired: 1 out]
    n41 = Index Array(array=w82, index #1=1 ("index"), index #2=7 ("index")) -> (element #1=w109:string, element #2=w108:string)
    "representation of cf" <- w109
    n42 = Index Array(array=w82, index #1=4 ("index"), index #2=1 ("index")) -> (element #1=w102:string, element #2=w103:string)
    n43 = String To Byte Array(string=w103) -> (unsigned byte array=w75:u8[])
    n44 = String To Byte Array(string=w102) -> (unsigned byte array=w94:u8[])
    n45 = String To Byte Array(string=w109) -> (unsigned byte array=w89:u8[])
    n46 = String To Byte Array(string=w108) -> (unsigned byte array=w106:u8[])
    n47 = for {
      tunnel: w75 -> [w141]
      tunnel: w94 -> [w140] mode=indexing
      tunnel: [w140] -> w93 mode=indexing if=w139
      n48 = Search 1D Array(1D array=w141, element=w140) -> (index of element=w143:i32)  [unwired: 1 in]
      n49 = Equal?(x=w143, y=-1) -> (x = y?=w139:bool)
    }
    n50 = for {
      tunnel: w89 -> [w146]
      tunnel: w106 -> [w145] mode=indexing
      tunnel: [w145] -> w71 if=w144
      n51 = Search 1D Array(1D array=w146, element=w145) -> (index of element=w148:i32)  [unwired: 1 in]
      n52 = Equal?(x=w148, y=-1) -> (x = y?=w144:bool)
    }
    n53 = Index Array(array=w82, index=8) -> (element=w99:string)
    n54 = String To Byte Array(string=w99) -> (unsigned byte array=w95:u8[])
    n55 = Build Array(w71) -> (w72:u8[])
    n56 = Build Array (concatenate)(w71, w93, w75) -> (w96:u8[])
    n57 = Byte Array To String(unsigned byte array=w93) -> (string=→"representation of bd":string)
    n58 = Byte Array To String(unsigned byte array=w72) -> (string=→"representation of a":string)
    n59 = for {
      tunnel: w96 -> [w136]
      tunnel: w95 -> [w135] mode=indexing
      tunnel: [w135] -> w98 mode=indexing if=w134
      n60 = Search 1D Array(1D array=w136, element=w135) -> (index of element=w138:i32)  [unwired: 1 in]
      n61 = Equal?(x=w138, y=-1) -> (x = y?=w134:bool)
    }
    n62 = Byte Array To String(unsigned byte array=w98) -> (string=→"representation of eg":string)
    n63 = for {
      tunnel: w92 -> [w133] mode=indexing
      tunnel: [w132] -> w90 mode=indexing
      n64 = String To Byte Array(string=w133) -> (unsigned byte array=w132:u8[])
    }
    n65 = Index Array(array=w89) -> (element #1=w88:u8, element #2=w87:u8)  [unwired: 2 in]
    n66 = for {
      tunnel: w90 -> [w119] mode=indexing
      tunnel: w88 -> [w124]
      tunnel: w87 -> [w125]
      tunnel: [w129] -> w80 if=w122
      tunnel: [w126] -> w79 if=w122
      tunnel: [w123] -> w77 if=w122
      tunnel: w71 -> [_]
      n67 = Search 1D Array(1D array=w119, element=w124) -> (index of element=w128:i32)  [unwired: 1 in]
      n68 = Search 1D Array(1D array=w119, element=w125) -> (index of element=w127:i32)  [unwired: 1 in]
      n69 = Equal?(x=w128, y=-1) -> (x = y?=w120:bool)
      n70 = Equal?(x=w127, y=-1) -> (x = y?=w121:bool)
      n71 = Or(x=w120, y=w121) -> (x .or. y?=w122:bool)
      n72 = Byte Array To String(unsigned byte array=w119) -> (string=w129:string)
      n73 = Select(t=w124, s=w120, f=w125) -> (s? t:f=w126:u8)
      n74 = Select(t=w125, s=w120, f=w124) -> (s? t:f=w123:u8)
    }
    "6" <- w80
    n75 = Build Array(w79) -> (w74:u8[])
    n76 = Build Array(w77) -> (w73:u8[])
    n77 = Byte Array To String(unsigned byte array=w74) -> (string=→"the letter it doesn't have is c":string)
    n78 = Byte Array To String(unsigned byte array=w73) -> (string=→"and the other is f":string)
    n79 = Replace Array Subset(array=w84, new element=TRUE, index=w81) -> (w85:bool[])
    n80 = Replace Array Subset(array=w82, new element=w80, index=w81) -> (w83:string[])
    n81 = Build Array(w74, w73, w72) -> ()  [unwired: 1 out]
  }
  "tally of digits (index is digit)" <- w19
  "representation of digit (index is digit)" <- w12
  "5 digits long" <- w7
  "6 digits long" <- w6
  "Found? (index is digit)" <- w2
  n82 = for {
    N: 7 -> [_]
    tunnel: [w174] -> w16 mode=indexing
    i -> [w177]
    # "Ascii 'a'"
    n83 = To Unsigned Byte Integer(number=w177) -> (unsigned 8bit integer=w175:u8)
    n84 = Add(x=w175, y=u8 97 ("x")) -> (x+y=w172:u8)
    n85 = Build Array(w172) -> (w173:u8[])
    n86 = Byte Array To String(unsigned byte array=w173) -> (string=w174:string)
  }
  "0=a,1=b etc" <- w16
  n87 = Add Array Elements(numeric array=w19) -> (sum=→"sum":i32)
